vi "MT Format Trellis Diagram.vi"(0 "waveform":T1={"t0"=0.0, "dt"=1.0, "Y"=[]} {"Y" format="%.3f"; "dt" format="%^.2e"; "t0" format="%.4f"}, 1 "trellis reference":refnum<vi>, 5 "symbol rate (Hz)":dbl=1.0 format="%.2f", 7 "trellis length":i32=2, 9 "modulation index":dbl=0.5 format="%.2f", 11 "error in (no error)":errorcluster, 12 "autoscale":bool) -> (4 "trellis diagram":cluster{"t0":dbl, "dt":dbl, "phase":dbl[]}[](array[cluster]) {"phase" format="%.2f"; "dt" format="%.2f"; "t0" format="%.2f"}, 15 "error out":errorcluster)   [LabVIEW 2020, in "niDMT.lvlib"]
doc: "Receives a complex-valued waveform, divides it into segments of (<B>trellis length</B> / <B>symbol rate</B>), and displays those segments as a <B>trellis diagram</B> on a standard LabVIEW waveform graph referenced by the <B>trellis reference</B> parameter."
uses:
  <vilib>/addons/Modulation/niDMT.lvlib
  <vilib>/addons/Modulation/Analog/controls/Complex Data Waveform.ctl
  <vilib>/addons/Modulation/Digital/General/subVIs/mod_Segment Array(real).vi
  <vilib>/Analysis/NI_AALPro.lvlib
  <vilib>/addons/Modulation/niAMT.lvlib
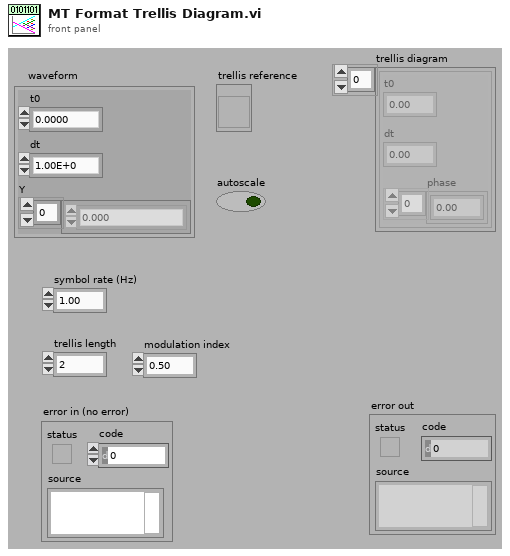
[diagram p1: front panel]
types:
  T1 = typedef "niAMT.lvlib/Complex Data Waveform.ctl" = cluster{"t0":dbl, "dt":dbl, "Y":cdb[]}
  T2 = cluster{dbl, "Numeric":dbl, "Unwrapped Phase":dbl[]}
  T3 = cluster{dbl, "Numeric":dbl, "Unwrapped Phase":dbl[]}[]
  T4 = cluster{"t0":dbl, "dt":dbl, "Unwrapped Phase":dbl[]}
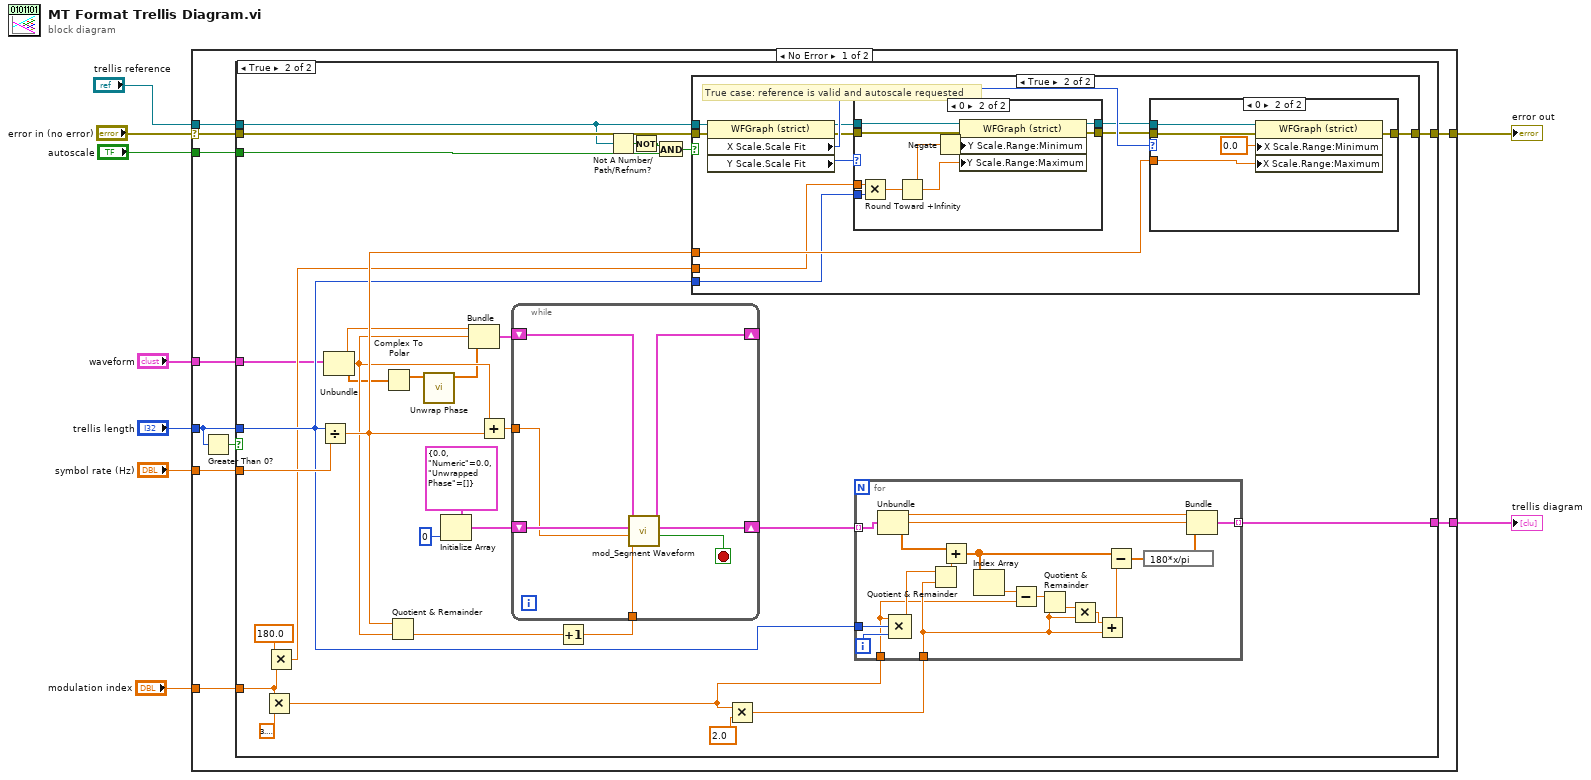
[diagram p0: block diagram]
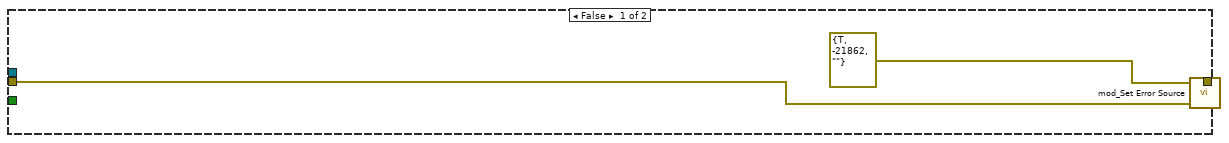
[diagram p2: hidden frame]
diagram:
  n1 = case shown="No Error" "error in (no error)" {
    selector: "error in (no error)" -> [w15 w111]
    tunnel: "symbol rate (Hz)" -> [w19 _]
    tunnel: "waveform" -> [w14 _]
    tunnel: [w18 _] -> w7
    tunnel: "autoscale" -> [w17 _]
    tunnel: "trellis length" -> [w11 _]
    tunnel: [w16 w111] -> w4
    tunnel: "modulation index" -> [w13 _]
    tunnel: "trellis reference" -> [w10 _]
    frame No Error {
      n2 = Greater Than 0?(x=w11) -> (x > 0?=w12:bool)
      n3 = case shown="True" w12 {
        tunnel: w19 -> [_ w54]
        tunnel: [_ w28] -> w18
        tunnel: w17 -> [_ w26]
        tunnel: [w22 w45] -> w16
        tunnel: w15 -> [w20 w44]
        tunnel: w11 -> [_ w43]
        tunnel: w14 -> [_ w29]
        tunnel: w13 -> [_ w33]
        tunnel: w10 -> [_ w23]
        frame False {
          n4 = call <vilib>:"mod_Set Error Source.vi"("initial error in (no error)"=w20, "final error in (no error)"=errorcluster {"status"=TRUE, "code"=-21862, "source"=""}) -> ("error out"=w22:errorcluster)  [unwired: 3 out]
        }
        frame True {
          n5 = Multiply(x=w33, y=3.141592653589793) -> (x*y=w30:dbl)
          n6 = Multiply(x=180.0, y=w33) -> (x*y=w31:dbl)
          n7 = Divide(x=w43, y=w54) -> (x/y=w46:dbl)
          n8 = Unbundle(w29) -> ("t0"=w42:dbl, "dt"=w41:dbl, "Y"=w40:cdb[])
          n9 = Complex To Polar(r * e^(i*theta)=w40) -> (theta=w37:dbl[])  [unwired: 1 out]
          n10 = Quotient & Remainder(x=w46, y=w41) -> (floor(x/y)=w51:dbl)  [unwired: 1 out]
          n11 = call <vilib>:"Unwrap Phase.vi"("Phase"=w37) -> ("Unwrapped Phase"=w39:dbl[])  [unwired: 1 in, 9 out]
          n12 = Initialize Array(T2 {0.0, "Numeric"=0.0, "Unwrapped Phase"=[]} ("output cluster"), 0 ("dimension size")) -> (w48:T3)
          n13 = Bundle("t0"=w42, "dt"=w41, "Unwrapped Phase"=w39) -> (w38:T4)  [unwired: 1 out]
          n14 = Add(x=w41, y=w46) -> (x+y=w50:dbl)
          n15 = Increment(x=w51) -> (x+1=w47:dbl)
          n16 = while {
            tunnel: w50 -> [w108]
            shift-right: [w104] -> w49
            shift-left: w48 -> [w109]
            shift-right: [w105] -> _
            shift-left: w38 -> [w110]
            tunnel: w47 -> [w107]
            stop <- w106 stop-if-true
            n17 = call-poly <vilib>:"mod_Segment Waveform.vi"("min samples per segment"=w107, "segment time"=w108, "graphs in"=w109, "waveform"=w110) -> ("done?"=w106:bool, "graphs out"=w104:cluster{dbl, "dt":dbl, dbl[]}[], "waveform out"=w105:cluster{"t0":dbl, "dt":dbl, "Y":dbl[]})  [unwired: 5 out]
          }
          n18 = Not A Number/Path/Refnum?(number/path/refnum=w23) -> (NaN/Path/Refnum?=w25:bool)
          n19 = Not(x=w25) -> (.not. x?=w27:bool)
          n20 = And(x=w27, y=w26) -> (x .and. y?=w24:bool)
          n21 = case shown="True" w24 {
            tunnel: w46 -> [_ w67]
            tunnel: [w55 w66] -> w45
            tunnel: w44 -> [w55 w64]
            tunnel: w43 -> [_ w56]
            tunnel: w31 -> [_ w57]
            tunnel: w23 -> [_ w65]
            frame False {
            }
            frame True {
              # "True case: reference is valid and autoscale requested"
              n22 = property class="WFGraph (strict)"(reference=w65, error in=w64) -> (reference out=w61:refnum<vi>, error out=w62:errorcluster, "X Scale.Scale Fit"=w63:u8, "Y Scale.Scale Fit"=w58:u8)
              n23 = case shown="0" w58 {
                tunnel: [w69 w78] -> w59
                tunnel: w56 -> [_ w77]
                tunnel: w57 -> [_ w76]
                tunnel: w61 -> [w68 w72]
                tunnel: w62 -> [w69 w71]
                tunnel: [w68 w70] -> w60
                frame 1, Default {
                }
                frame 0 {
                  n24 = Multiply(x=w76, y=w77) -> (x*y=w74:dbl)
                  n25 = Round Toward +Infinity(x=w74) -> (ceil(x): smallest int >= x=w73:dbl)
                  n26 = Negate(x=w73) -> (-x=w75:dbl)
                  n27 = property class="WFGraph (strict)"(reference=w72, error in=w71, "Y Scale.Range:Minimum"=w75, "Y Scale.Range:Maximum"=w73) -> (reference out=w70:refnum<vi>, error out=w78:errorcluster)
                }
              }
              n28 = case shown="0" w63 {
                tunnel: w67 -> [_ w84]
                tunnel: [w79 w83] -> w66
                tunnel: w60 -> [_ w81]
                tunnel: w59 -> [w79 w80]
                frame 1, Default {
                }
                frame 0 {
                  n29 = property class="WFGraph (strict)"(reference=w81, error in=w80, "X Scale.Range:Minimum"=0.0, "X Scale.Range:Maximum"=w84) -> (error out=w83:errorcluster)  [unwired: 1 out]
                }
              }
            }
          }
          n30 = Multiply(x=w30, y=2.0) -> (x*y=w34:dbl)
          n31 = for {
            tunnel: w49 -> [w103] mode=indexing
            tunnel: [w100] -> w28 mode=indexing
            tunnel: w43 -> [w99]
            tunnel: w34 -> [w88]
            tunnel: w30 -> [w86]
            i -> [w98]
            n32 = Unbundle(w103) -> (w102:dbl, "Numeric"=w101:dbl, "Unwrapped Phase"=w89:dbl[])
            n33 = Compound Arithmetic op=MULTIPLY(w86, w99, w98) -> (w94:dbl)
            n34 = Quotient & Remainder(x=w94, y=w88) -> (x-y*floor(x/y)=w97:dbl)  [unwired: 1 out]
            n35 = Add(x=w89, y=w97) -> (x+y=w93:dbl[])
            n36 = Index Array(array=w93) -> (element=w96:dbl)  [unwired: 1 in]
            n37 = Subtract(x=w96, y=w86) -> (x-y=w92:dbl)
            n38 = Quotient & Remainder(x=w92, y=w88) -> (floor(x/y)=w95:dbl)  [unwired: 1 out]
            n39 = Multiply(x=w95, y=w88) -> (x*y=w91:dbl)
            n40 = Add(x=w91, y=w88) -> (x+y=w90:dbl)
            n41 = Subtract(x=w93, y=w90) -> (x-y=w87:dbl[])
            n42 = expression code="180*x/pi"(w87) -> (w85:dbl[])
            n43 = Bundle(w102, "Numeric"=w101, w85) -> (w100:cluster{dbl, "Numeric":dbl, dbl[]})  [unwired: 1 out]
          }
        }
      }
    }
    frame Error {
    }
  }
  "trellis diagram" <- w7
  "error out" <- w4
